vi "soma_diferenca.vi"(8 "Slide 2":i8(slide) scale=0.0..10.0, 11 "Slide":i8(slide) scale=0.0..10.0) -> (0 "A-B":dbl(knob) scale=-10.0..10.0, 3 "A+B":dbl(knob) scale=0.0..20.0)   [LabVIEW 2025]
panel:
  out "Counter":i32
  in  "stop":bool
  out "Product":dbl(knob) scale=-3000.0..1100.0
  in  "Boolean (down=0)":bool
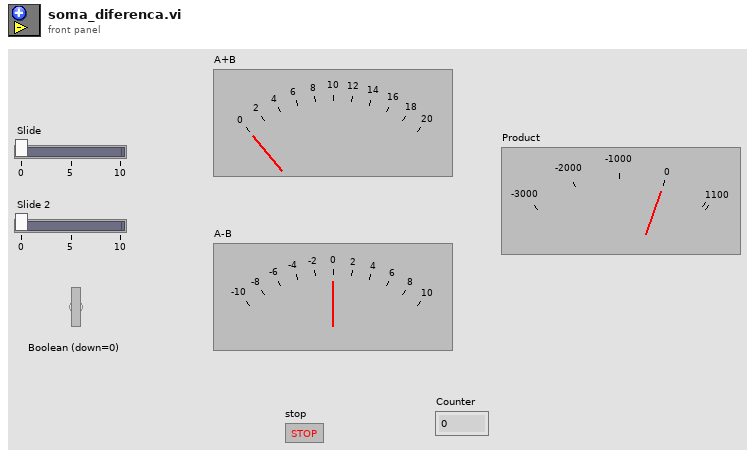
[diagram p1: front panel]
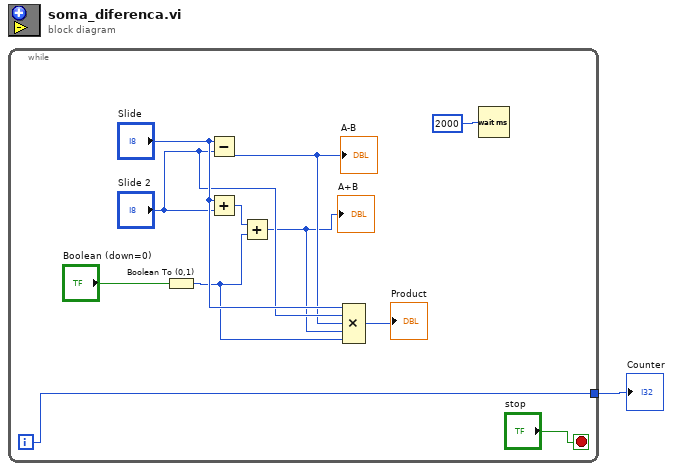
[diagram p0: block diagram]
diagram:
  n1 = while {
    tunnel: [w3] -> w1
    i -> [w3]
    stop <- "stop" stop-if-true
    n2 = Boolean To (0,1)(Boolean="Boolean (down=0)") -> (0, 1=w6:i16)
    n3 = Subtract(x="Slide", y="Slide 2") -> (x-y=w8:i8)
    "A-B" <- w8
    n4 = Add(x="Slide", y="Slide 2") -> (x+y=w12:i8)
    n5 = Add(x=w12, y=w6) -> (x+y=w7:i16)
    "A+B" <- w7
    n6 = Compound Arithmetic op=MULTIPLY("Slide", "Slide 2", w8, w7, w6) -> (→"Product":i16)
    n7 = Wait (ms)(milliseconds to wait=u32 2000) -> ()  [unwired: 1 out]
  }
  "Counter" <- w1
